vi "Log_StringClass.vi"(10 "Message":refnum<class "Abs_String.lvclass">, 11 "EventLog":refnum<class "abs_EventLog.lvclass">) -> (3 "node out":refnum<class "bt_Log.lvclass">)   [LabVIEW 2021, in "BT.lvlib"]
uses:
  BT.lvlib
  Nodes/Leaves/Log/bt_Log.lvclass
  <vilib>/TSA/Event Log/abs_EventLog/abs_EventLog.lvclass
  <vilib>/TSA/Abstract Data Classes/Abs_Types/String/Abs_String.lvclass
  Nodes/Leaves/Log/bt_Log.lvclass/bt_Log.ctl
  Nodes/Leaves/Log/Properties/Write EventLog.vi
  Nodes/Leaves/Log/Properties/Write Message.vi
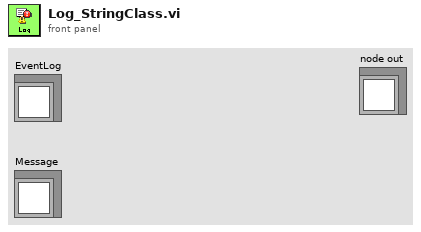
[diagram p1: front panel]
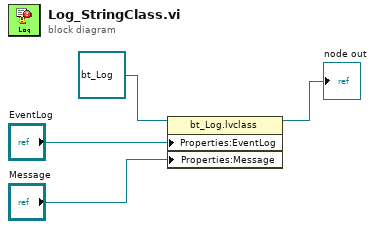
[diagram p0: block diagram]
diagram:
  n1 = property class="bt_Log.lvclass"(reference=refnum<class "bt_Log.lvclass"> refnum ("BT.lvlib:bt_Log.lvclass"), "Properties:EventLog"="EventLog", "Properties:Message"="Message") -> (reference out=→"node out":refnum<class "bt_Log.lvclass">)  [unwired: 1 in, 1 out]
